vi "Build Variable Definition Array.vi"(6 "Start Dest Index":i32, 8 "Error In":errorcluster, 9 "Array of Variable Indices":i32[](array[numeric]), 10 "Variable":string, 11 "Formula String":string) -> (0 "Error Out":errorcluster, 2 "Definition Array":T1[](array[typedef]), 3 "Formula String (with renamed variables)":string, 4 "New Variable Names":string[](array[string]), 5 "Ordered Original Variable Names":string[](array[string]))   [LabVIEW 2021, in "Formula.lvlib"]
uses:
  Formula.lvlib
  Binary Formula.ctl
  Binary Formula Step.ctl
  Binary Operator.ctl
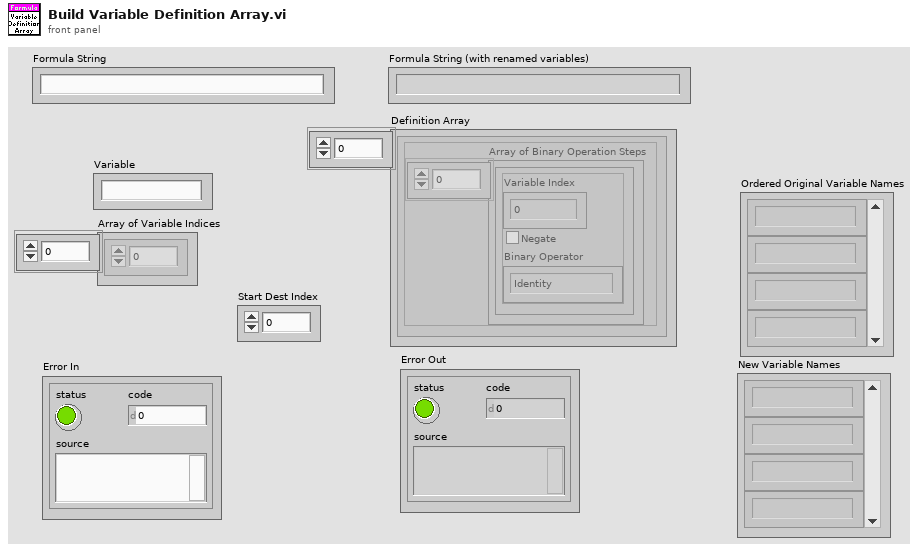
[diagram p1: front panel]
types:
  T1 = typedef "Formula.lvlib/Binary Formula.ctl" = cluster{"Array of Binary Operation Steps":T2[]}
  T2 = typedef "Formula.lvlib/Binary Formula Step.ctl" = cluster{"Variable Index":i32, "Negate":bool, "Binary Operator":T3}
  T3 = typedef "Formula.lvlib/Binary Operator.ctl" = enum16{"Identity", "AND", "OR"}
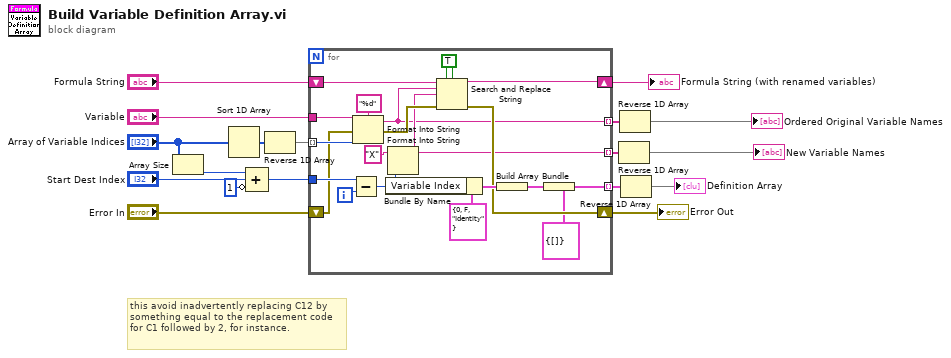
[diagram p0: block diagram]
diagram:
  # "this avoid inadvertently replacing C12 by something equal to the replacement code for C1 followed by 2, for instance."
  n1 = Array Size(array="Array of Variable Indices") -> (size(s)=w5:i32)
  n2 = Sort 1D Array(array="Array of Variable Indices") -> (sorted array=w17:i32[])
  n3 = Compound Arithmetic op=ADD(w5, "Start Dest Index", invert 1 ("value")) -> (w7:i32)
  n4 = Reverse 1D Array(array=w17) -> (reversed array=w14:i32[])
  n5 = for {
    tunnel: w14 -> [w32] mode=indexing
    tunnel: w7 -> [w38]
    tunnel: [w19] -> w8 mode=indexing
    shift-right: [w30] -> w12
    shift-left: "Formula String" -> [w31]
    tunnel: "Variable" -> [w34]
    shift-right: [w26] -> w11
    shift-left: "Error In" -> [w27]
    tunnel: [w23] -> w9 mode=indexing
    tunnel: [w22] -> w10 mode=indexing
    i -> [w37]
    w29 = TRUE ("replace all? (F)")
    n6 = Subtract(x=w38, y=w37) -> (x-y=w25:i32)
    n7 = Format Into String(format string="%d", initial string=w34, error in=w27, w32) -> (resulting string=w22:string, error out=w28:errorcluster)
    n8 = Bundle By Name(cluster=T2 {"Variable Index"=0, "Negate"=FALSE, "Binary Operator"=enum."Identity"} ("Binary Operation Step"), "Variable Index"=w25) -> (w35:T2)
    n9 = Format Into String(initial string="X", w25) -> (resulting string=w23:string)  [unwired: 2 in, 1 out]
    n10 = Search and Replace String(replace all?=w29, case sensitive?=w29, input string=w31, search string=w22, replace string=w23, error in=w28) -> (result string=w30:string, error out=w26:errorcluster)  [unwired: 2 in, 2 out]
    n11 = Build Array(w35) -> (w21:T2[])
    n12 = Bundle(cluster=T1 {"Array of Binary Operation Steps"=[]} ("Binary Formula"), "Array of Binary Operation Steps"=w21) -> (w19:T1)
  }
  "Error Out" <- w11
  "Formula String (with renamed variables)" <- w12
  n13 = Reverse 1D Array(array=w9) -> (reversed array=→"New Variable Names":string[])
  n14 = Reverse 1D Array(array=w10) -> (reversed array=→"Ordered Original Variable Names":string[])
  n15 = Reverse 1D Array(array=w8) -> (reversed array=→"Definition Array":T1[])
